vi "DigitalInput-Daemon.vi"(3 "error in":errorcluster, 4 "References":T2, 5 "Configuration":T3) -> (0 "error out":errorcluster)   [LabVIEW 2011]
doc: "Input driver for digital input lines.\n\nThis daemon runs at a specified rate using a wait() inside a while loop. On each update, it reads the inputs (DAQmx lines) and writes it to the data cluster. It also checks to see if Stop is true, in which case it exits the while loop and shuts down.\n\n\"Configuration\" is a cluster containing \"Lines\" (an array of DAQmx lines) and \"Refresh period (ms)\" (which is wired to the wait() inside the while loop).\n\n\"References\" is a struct containing \"semaphore\" (a semaphore reference used to protect access to the data cluster), \"Data Refnum\" (a reference to the data cluster that this daemon will update), and \"Stop Refnum\" ( reference to the boolean control that can stop this daemon)."
uses:
  DigitalInput-Configuration.ctl
  <vilib>/DAQmx/create/channels.llb/DAQmx Create Channel (DI-Digital Input).vi
panel:
  # "This VI goes into a while loop\nthat updates Data Refnum\n(protected by a semaphore)\nuntil stopped by Stop Refnum.\n\nIt is designed to be called\nasynchronously."
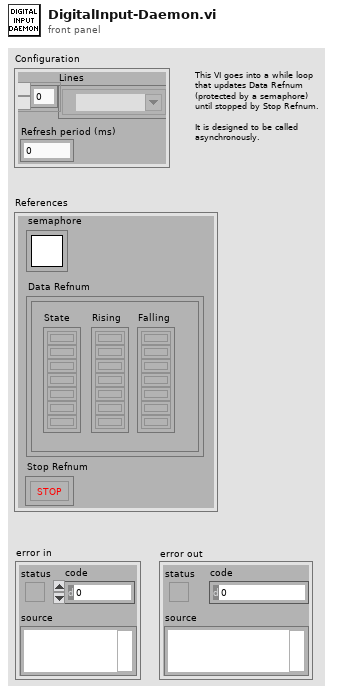
[diagram p1: front panel]
types:
  T1 = typedef "Semaphore RefNum" = refnum<k1>
  T2 = cluster{"Stop Refnum":refnum<vi>, "Data Refnum":refnum<vi>, "semaphore":T1}
  T3 = typedef "DigitalInput-Configuration.ctl" = cluster{"Lines":tag[], "Refresh period (ms)":u32}
  T4 = cluster{"State":bool[], "Rising":bool[], "Falling":bool[]}
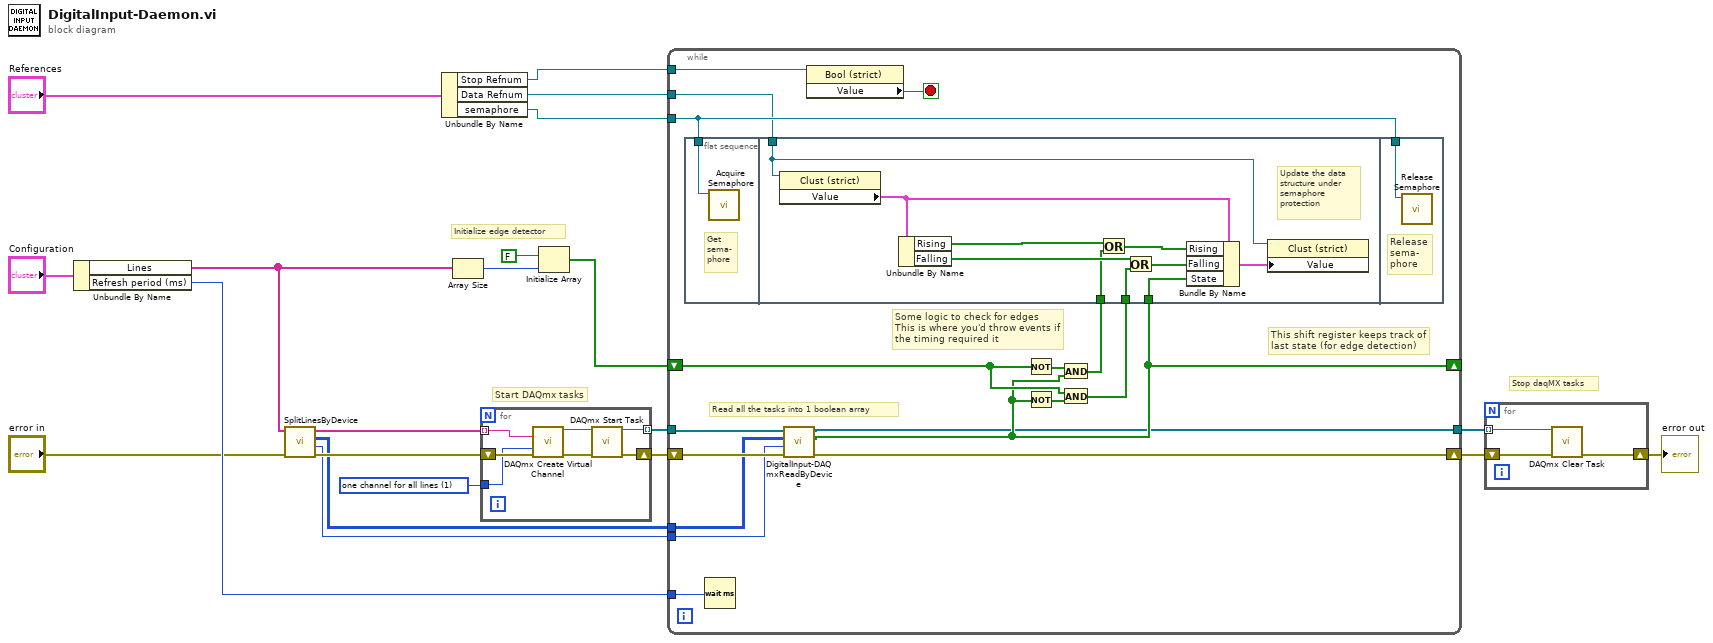
[diagram p0: block diagram]
diagram:
  w7 = 1 items=["one channel for each line", "one channel for all lines"] ("line grouping")
  # "Start DAQmx tasks"
  # "Initialize edge detector"
  # "Stop daqMX tasks"
  n1 = Unbundle By Name("Configuration") -> ("Lines"=w5:tag[], "Refresh period (ms)"=w17:u32)
  n2 = call "SplitLinesByDevice.vi"("error in"="error in", "Lines"=w5) -> ("error out"=w8:errorcluster, "Num lines"=w1:i32, "Original indices"=w2:i32[][], "Lines by device"=w9:string[])  [unwired: 6 in]
  n3 = Unbundle By Name("References") -> ("Stop Refnum"=w13:refnum<vi>, "Data Refnum"=w14:refnum<vi>, "semaphore"=w15:T1)
  n4 = Array Size(array=w5) -> (size(s)=w18:i32)
  n5 = for {
    tunnel: w9 -> [w28] mode=indexing
    tunnel: w7 -> [w26]
    shift-right: [w24] -> w4
    shift-left: w8 -> [w27]
    tunnel: [w22] -> w3 mode=indexing
    n6 = call-poly <vilib>:"DAQmx Create Virtual Channel.vi"("lines"=w28, "line grouping"=w26, "error in"=w27) -> ("task out"=w23:refnum<k21>, "error out"=w25:errorcluster)  [unwired: 11 in]
    n7 = call <vilib>:"DAQmx Start Task.vi"("task/channels in"=w23, "error in"=w25) -> ("task out"=w22:refnum<k21>, "error out"=w24:errorcluster)  [unwired: 12 in]
  }
  n8 = Initialize Array(FALSE ("Value"), w18) -> (w20:bool[])
  n9 = while {
    tunnel: w15 -> [w43]
    tunnel: w17 -> [w44]
    tunnel: w14 -> [w42]
    shift-right: [w33] -> _
    shift-left: w20 -> [w41]
    tunnel: w13 -> [w36]
    shift-right: [w34] -> w12
    shift-left: w4 -> [w35]
    tunnel: [w32] -> w10
    tunnel: w3 -> [w31]
    tunnel: w2 -> [w30]
    tunnel: w1 -> [w29]
    stop <- w45 stop-if-true
    # "Read all the tasks into 1 boolean array"
    # "This shift register keeps track of \nlast state (for edge detection)"
    # "Some logic to check for edges\nThis is where you'd throw events if\nthe timing required it"
    n10 = flat-sequence {
      tunnel: w43 -> [w46]
      tunnel: w42 -> [w56]
      tunnel: w33 -> [w49]
      tunnel: w38 -> [w48]
      tunnel: w37 -> [w47]
      tunnel: w43 -> [w57]
      frame #0 {
        # "Get \nsema-\nphore"
        n11 = call <vilib>:"Acquire Semaphore.vi"("semaphore"=w46) -> ()  [unwired: 4 in, 3 out]
      }
      frame #1 {
        # "Update the data\nstructure under\nsemaphore\nprotection"
        n12 = property class="Clust (strict)"(reference=w56) -> ("Value"=w54:T4)  [unwired: 1 in, 2 out]
        n13 = Unbundle By Name(w54) -> ("Rising"=w53:bool[], "Falling"=w51:bool[])
        n14 = Or(x=w53, y=w48) -> (x .or. y?=w52:bool[])
        n15 = Or(x=w51, y=w47) -> (x .or. y?=w50:bool[])
        n16 = Bundle By Name(cluster=w54, "Rising"=w52, "Falling"=w50, "State"=w49) -> (w55:T4)
        n17 = property class="Clust (strict)"(reference=w56, "Value"=w55) -> ()  [unwired: 1 in, 2 out]
      }
      frame #2 {
        # "Release \nsema-\nphore"
        n18 = call <vilib>:"Release Semaphore.vi"("semaphore"=w57) -> ()  [unwired: 5 in, 2 out]
      }
    }
    n19 = Wait (ms)(milliseconds to wait=w44) -> ()  [unwired: 1 out]
    n20 = call "DigitalInput-DAQmxReadByDevice.vi"("error in"=w35, "Num lines"=w29, "Original indices"=w30, "Tasks by device"=w31) -> ("error out"=w34:errorcluster, "data"=w33:bool[], "Tasks (dup)"=w32:refnum<k21>[])  [unwired: 5 in]
    n21 = property class="Bool (strict)"(reference=w36) -> ("Value"=w45:bool)  [unwired: 1 in, 2 out]
    n22 = Not(x=w41) -> (.not. x?=w40:bool[])
    n23 = Not(x=w33) -> (.not. x?=w39:bool[])
    n24 = And(x=w40, y=w33) -> (x .and. y?=w38:bool[])
    n25 = And(x=w41, y=w39) -> (x .and. y?=w37:bool[])
  }
  n26 = for {
    tunnel: w10 -> [w58] mode=indexing
    shift-right: [w59] -> w11
    shift-left: w12 -> [w60]
    n27 = call <vilib>:"DAQmx Clear Task.vi"("task in"=w58, "error in"=w60) -> ("error out"=w59:errorcluster)  [unwired: 13 in]
  }
  "error out" <- w11
